vi "Trapezoid Position Converter.vi"(10 "Distance":dbl, 11 "Initial Parameter":enum16{"Position", "Trapezoid Distance"}(ring)) -> (3 "Transformed Distance":dbl)   [LabVIEW 2023]
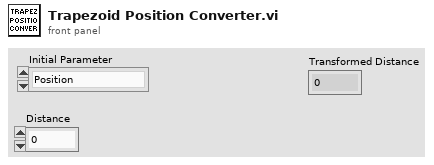
[diagram p1: front panel]
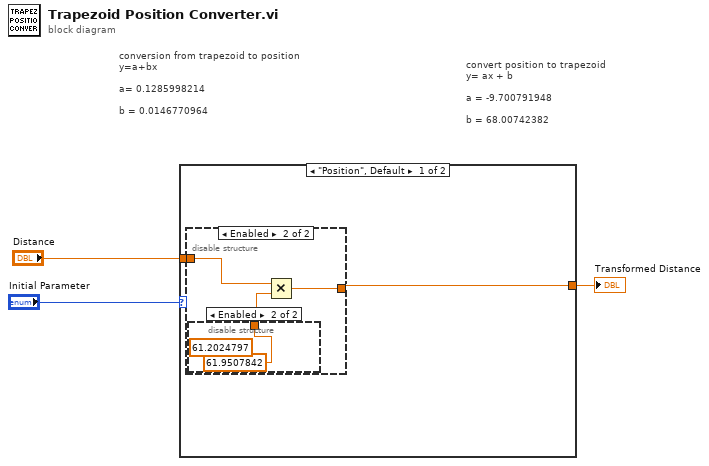
[diagram p0: block diagram]
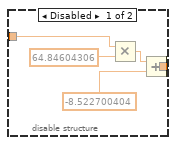
[diagram p2: hidden frame]
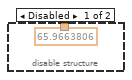
[diagram p3: hidden frame]
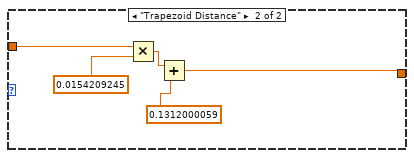
[diagram p4: hidden frame]
diagram:
  # "convert position to trapezoid\ny= ax + b\n\na = -9.700791948\n\nb = 68.00742382"
  # "conversion from trapezoid to position\ny=a+bx\n\na= 0.1285998214\n\nb = 0.0146770964"
  n1 = case shown="\"Position\", Default" "Initial Parameter" {
    tunnel: "Distance" -> [w5 w17]
    tunnel: [w4 w16] -> w1
    frame "Position", Default {
      n2 = disable-structure shown="Enabled" {
        disable-tunnel: w5 -> [w9 w12]
        disable-tunnel: [w6 w13] -> w4
        frame Disabled {
          n3 = Multiply(x=w9, y=64.84604306) -> (x*y=w10:dbl)
          n4 = Add(x=w10, y=-8.522700404) -> (x+y=w6:dbl)
        }
        frame Enabled {
          n5 = disable-structure shown="Enabled" {
            disable-tunnel: [65.9663806 ("y") 61.9507842 ("y")] -> w11
            frame Disabled {
            }
            frame Enabled {
              (unwired) 61.2024797 ("y")
            }
          }
          n6 = Multiply(x=w12, y=w11) -> (x*y=w13:dbl)
        }
      }
    }
    frame "Trapezoid Distance" {
      n7 = Multiply(x=w17, y=0.0154209245) -> (x*y=w20:dbl)
      n8 = Add(x=w20, y=0.1312000059) -> (x+y=w16:dbl)
    }
  }
  "Transformed Distance" <- w1
